vi "tcpLoop.vi"(8 "error in (no error)":errorcluster) -> (0 "error out":errorcluster)   [LabVIEW 2015]
panel:
  in  "Local Interface":string="10.10.20.1"
  out "remote port":u16
  out "Remote address":string
  in  "Local Port":u16=50000
  out "IMUvalues":dbl[](array[numeric])
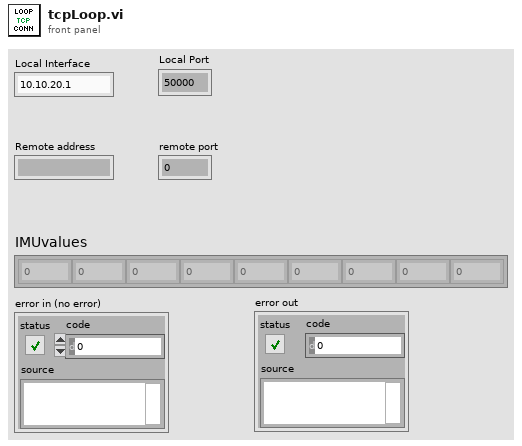
[diagram p1: front panel]
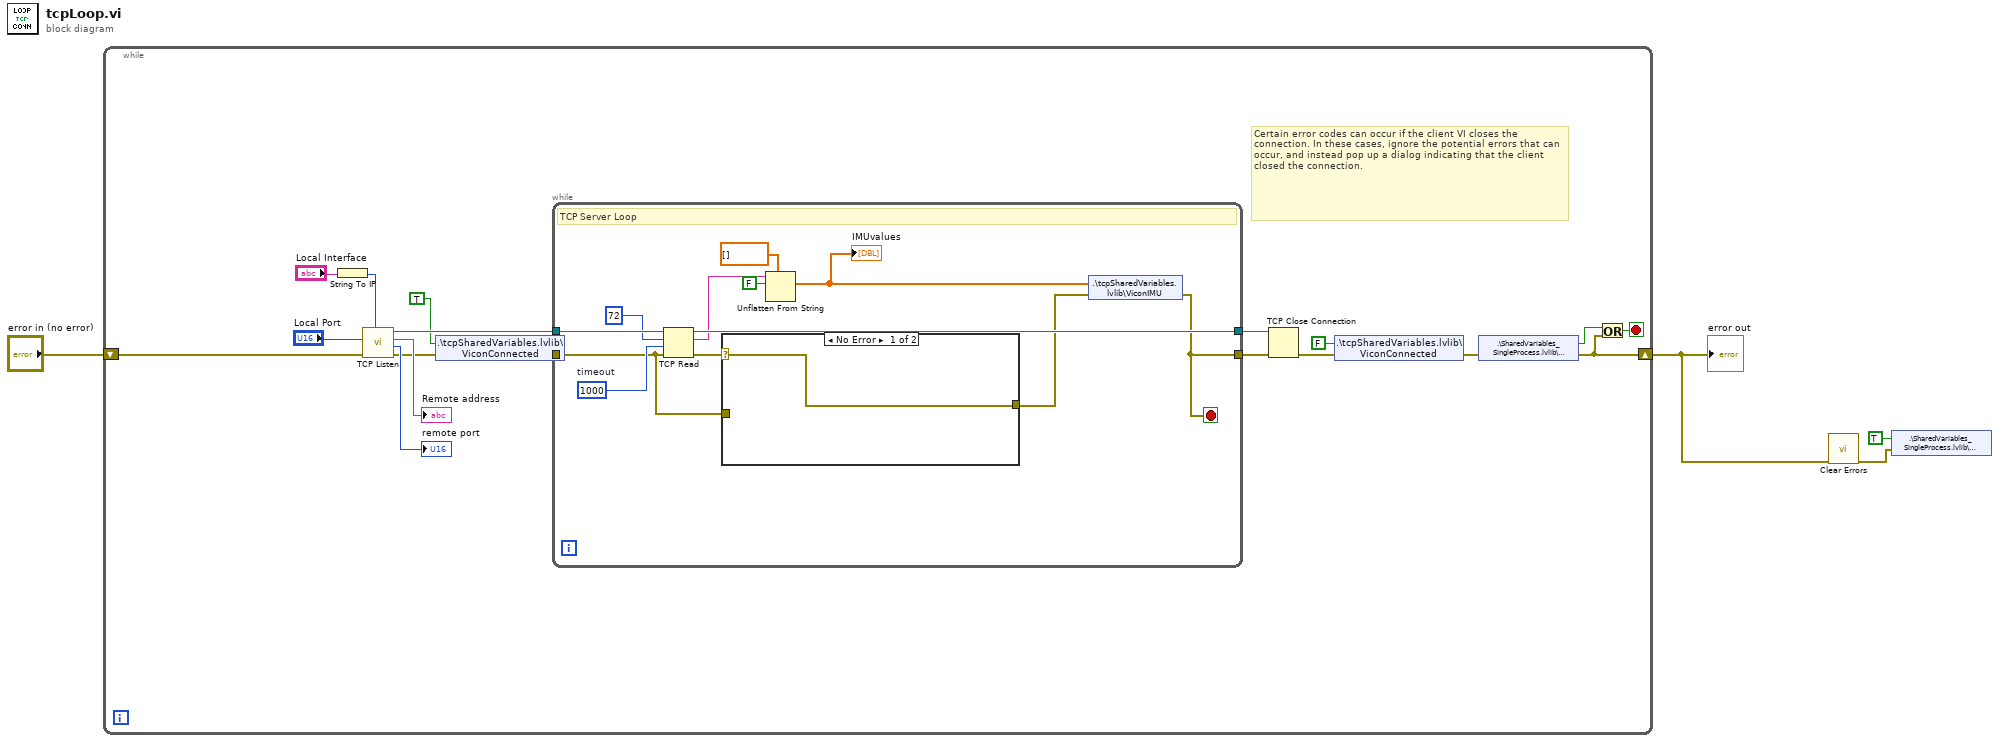
[diagram p0: block diagram]
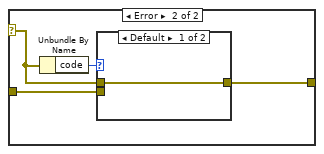
[diagram p2: hidden frame]
diagram:
  n1 = while {
    shift-right: [w5] -> w1
    shift-left: "error in (no error)" -> [w9]
    stop <- w6 stop-if-true
    # "Certain error codes can occur if the client VI closes the connection. In these cases, ignore the potential errors that can occur, and instead pop up a dialog indicating that the client closed the connection."
    n2 = String To IP(1:"Local Interface") -> (0:w16:u32)
    n3 = call <vilib>:"TCP Listen.vi"("net address"=w16, "error in (no error)"=w9, "port"="Local Port") -> ("error out"=w11:errorcluster, "remote port"=→"remote port":u16, "remote address"=→"Remote address":string, "connection ID"=w20:refnum<k5>)  [unwired: 4 in, 1 out]
    n4 = shared-variable ".\\tcpSharedVariables.lvlib\\ViconConnected"(TRUE ("Connected"), error in=w11) -> (error out=w10:errorcluster)
    n5 = while {
      tunnel: [w23] -> w21
      tunnel: [w34] -> w22
      tunnel: w20 -> [w31]
      tunnel: w10 -> [w30]
      stop <- w23 stop-if-true
      w33 = 1000  # timeout
      # "TCP Server Loop"
      n6 = TCP Read(connection ID=w31, bytes to read=72, error in (no error)=w30, 9:w33) -> (connection ID out=w34:refnum<k5>, data out=w28:string, error out=w32:errorcluster)  [unwired: 1 out]
      n7 = case shown="No Error" w32 {
        selector: w32 -> [w35 w38]
        tunnel: [w35 w36] -> w24
        tunnel: w30 -> [_ w37]
        frame No Error {
        }
        frame Error {
          n8 = Unbundle By Name(w38) -> ("code"=w39:i32)
          n9 = case shown="Default" w39 {
            tunnel: w38 -> [w40 _]
            tunnel: w37 -> [_ w41]
            tunnel: [w40 w41] -> w36
            frame Default {
            }
            frame 56 {
            }
          }
        }
      }
      n10 = Unflatten From String(type=dbl[] [] ("Waveform Graph 2"), binary string=w28, data includes array or string size? (T)=FALSE) -> (value=w25:dbl[])  [unwired: 2 in, 2 out]
      "IMUvalues" <- w25
      n11 = shared-variable ".\\tcpSharedVariables.lvlib\\ViconIMU"(w25, error in=w24) -> (error out=w23:errorcluster)
    }
    n12 = TCP Close Connection(connection ID=w22, error in (no error)=w21) -> (error out=w14:errorcluster)  [unwired: 2 out]
    n13 = shared-variable ".\\tcpSharedVariables.lvlib\\ViconConnected"(FALSE ("Connected"), error in=w14) -> (error out=w8:errorcluster)
    n14 = shared-variable ".\\SharedVariables_SingleProcess.lvlib\\GlobalStop"(error in=w8) -> (w7:bool, error out=w5:errorcluster)
    n15 = Or(x=w7, y=w5) -> (x .or. y?=w6:bool)
  }
  "error out" <- w1
  n16 = call <vilib>:"Clear Errors.vi"("error in (no error)"=w1) -> ("error out"=w2:errorcluster)  [unwired: 5 in, 1 out]
  n17 = shared-variable ".\\SharedVariables_SingleProcess.lvlib\\GlobalStop"(TRUE ("GlobalStop"), error in=w2) -> ()  [unwired: 1 out]
